vi "New.vi"(8 "error in (no error)":errorcluster, 11 "reference in":refnum<class "Component_Template.lvclass">) -> (0 "error out":errorcluster, 3 "reference out":refnum<class "Component_Template.lvclass">)   [LabVIEW 2022 SP3, in "Component_Template.lvlib" / "Component_Template.lvclass"]
uses:
  Component_Template.lvclass
  ObjectAttributes.ctl
  Config.ctl
  Component_Template.lvclass/Component_Template.ctl
  Components/ViPER.lvlibp/ViPER.lvclass
panel:
  in  "Data":T1
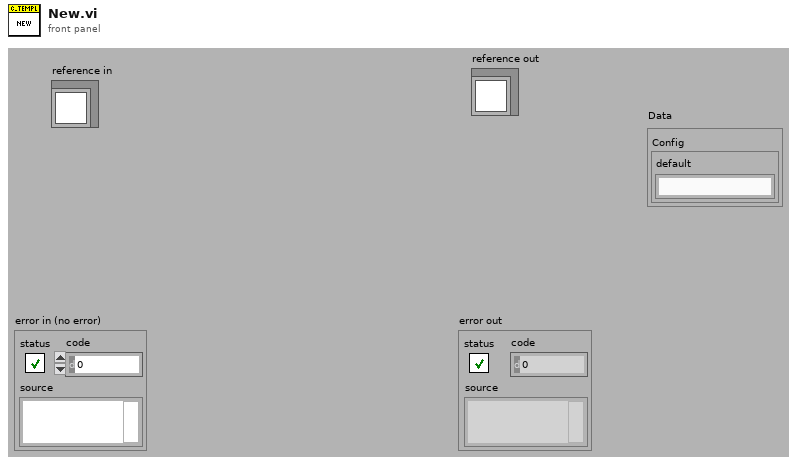
[diagram p1: front panel]
types:
  T1 = typedef "Component_Template.lvlib/Component_Template.lvclass/ObjectAttributes.ctl" = cluster{"Config":T2}
  T2 = typedef "Component_Template.lvlib/Component_Template.lvclass/Config.ctl" = cluster{"default":string}
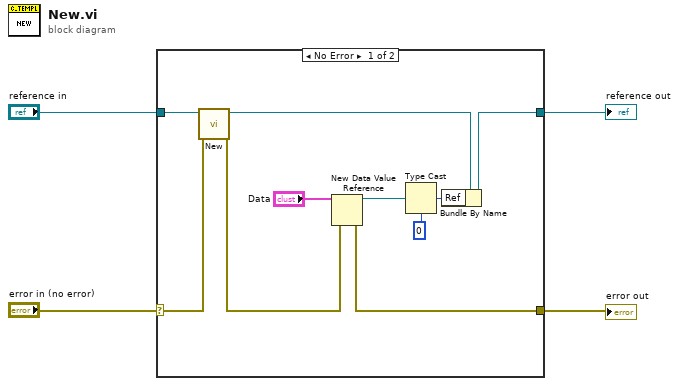
[diagram p0: block diagram]
diagram:
  n1 = case shown="No Error" "error in (no error)" {
    selector: "error in (no error)" -> [w7 w15]
    tunnel: "reference in" -> [w14 w16]
    tunnel: [w5 w15] -> w3
    tunnel: [w12 w16] -> w2
    frame No Error {
      n2 = call-parent "New.vi"("error in (no error)"=w7, "reference in"=w14) -> ("error out"=w6:errorcluster, "reference out"=w11:refnum<class "Component_Template.lvclass">)  [unwired: 8 in]
      n3 = New Data Value Reference(data value="Data", error in=w6) -> (data value reference=w9:refnum<data-value>, error out=w5:errorcluster)
      n4 = Type Cast(type=u32 0 ("DataRef"), x=w9) -> (*(type *) &x=w8:u32)
      n5 = Bundle By Name(cluster=w11, "Ref"=w8) -> (w12:refnum<class "Component_Template.lvclass">)
    }
    frame Error {
    }
  }
  "error out" <- w3
  "reference out" <- w2
